vi "Read Timing Source Type.vi"(8 "error in":errorcluster, 11 "Standard Engine Repo Data in":refnum<class "Standard Engine Configuration.lvclass">) -> (0 "error out":errorcluster, 2 "Timing Source":T1, 3 "Standard Engine Repo Data out":refnum<class "Standard Engine Configuration.lvclass">)   [LabVIEW 2013, in "Standard Engine Configuration.lvclass"]
uses:
  Standard Engine Configuration.lvclass
  Supported Timing Sources.ctl
  Standard Engine Configuration.lvclass/Standard Engine Configuration.ctl
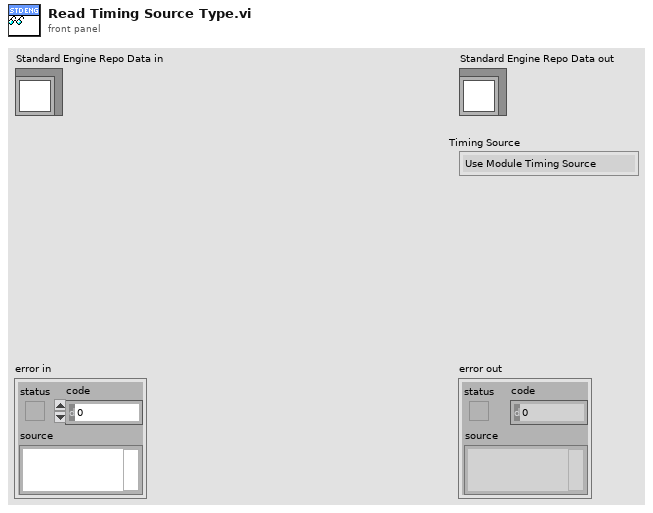
[diagram p1: front panel]
types:
  T1 = typedef "Standard Engine Configuration.lvclass/Supported Timing Sources.ctl" = enum16{"Use Module Timing Source", "1 kHz Clock", "1 MHz Clock", "Synchronize to Scan Engine"}
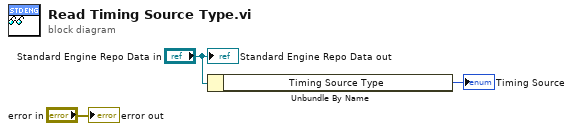
[diagram p0: block diagram]
diagram:
  n1 = Unbundle By Name("Standard Engine Repo Data in") -> ("Timing Source Type"=→"Timing Source":T1)
  "error out" <- "error in"
  "Standard Engine Repo Data out" <- "Standard Engine Repo Data in"
